vi "Find Component Configuration.vi"(8 "error in (no error)":errorcluster, 10 "component":string, 11 "configurations in":T1[](array[typedef])) -> (0 "error out":errorcluster, 1 "index":i32, 2 "component configuration":T1, 3 "configurations out":T1[](array[typedef]), 4 "found?":bool)   [LabVIEW 2019, in "DSF Core.lvlib"]
uses:
  DSF Core.lvlib
  Typedefs/DSF Component Configuration.ctl
  Typedefs/DSF Version Info.ctl
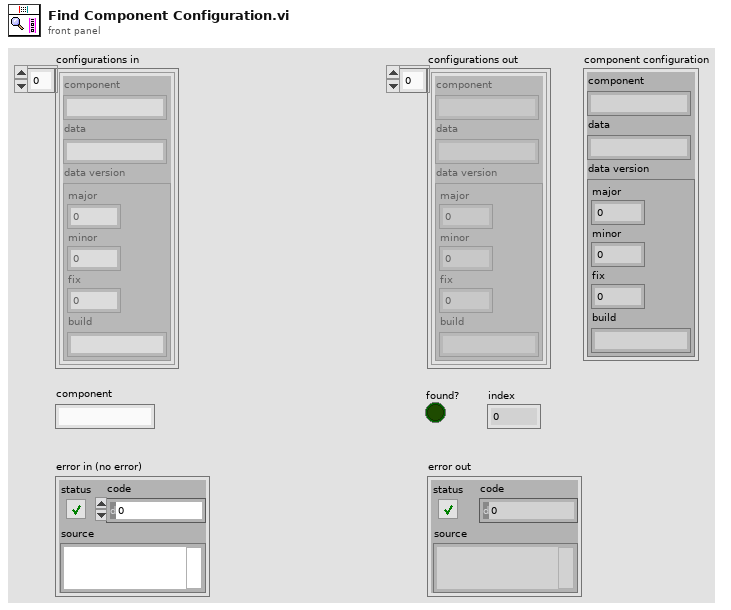
[diagram p1: front panel]
types:
  T1 = typedef "DSF Core.lvlib/DSF Component Configuration.ctl" = cluster{"component":string, "data":string, "data version":T2}
  T2 = typedef "DSF Core.lvlib/DSF Version Info.ctl" = cluster{"major":u32, "minor":u32, "fix":u32, "build":string}
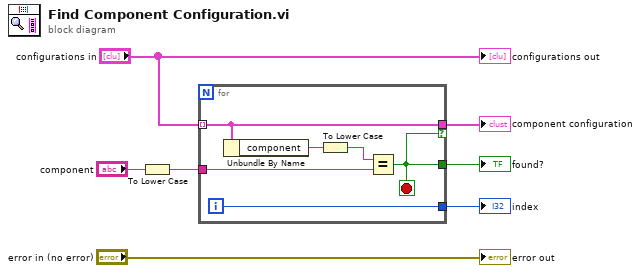
[diagram p0: block diagram]
diagram:
  n1 = To Lower Case(string="component") -> (all lower case string=w2:string)
  n2 = for {
    tunnel: "configurations in" -> [w13] mode=indexing
    tunnel: [w13] -> w6 if=w11
    tunnel: w2 -> [w12]
    tunnel: [w11] -> w5
    tunnel: [w8] -> w1
    i -> [w8]
    stop <- w11 stop-if-true
    n3 = Unbundle By Name(w13) -> ("component"=w9:string)
    n4 = To Lower Case(string=w9) -> (all lower case string=w10:string)
    n5 = Equal?(x=w10, y=w12) -> (x = y?=w11:bool)
  }
  "component configuration" <- w6
  "found?" <- w5
  "index" <- w1
  "error out" <- "error in (no error)"
  "configurations out" <- "configurations in"
